vi "Meas_monitordata_struct_Add.vi"(1 "Active Sensors":bool[](array[boolean]), 2 "chk2scan":bool, 5 "Controls[]":refnum<vi>[](array[refnum]), 7 "Meas_monitordata_struct输入":refnum<k24>[](array[refnum]), 11 "错误输入（无错误）":errorcluster, 12 "sweep_count":i32, 13 "Meas_rang":i32[](array[numeric])) -> (6 "Meas_monitordata_struct输出":refnum<k24>[](array[refnum]), 15 "错误输出":errorcluster)   [LabVIEW 2017]
doc: "for measurement monitor data"
uses:
  D:/test/PDLSTS/LV_PDL_Sample/DLL/STSProcess.dll
  DLL/STSProcess.dll
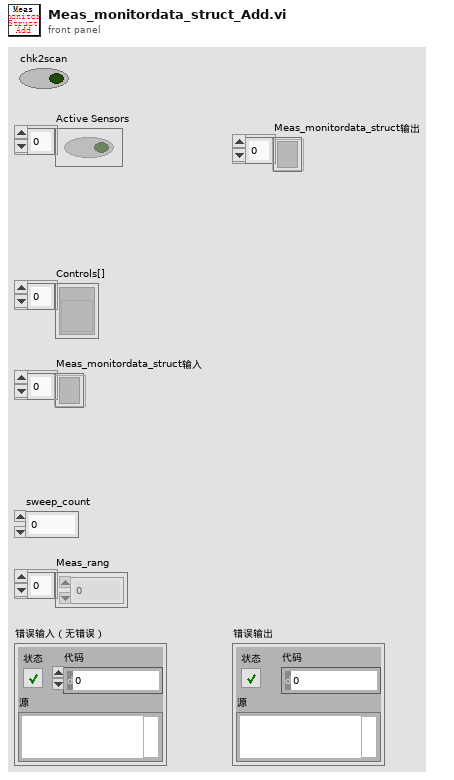
[diagram p1: front panel]
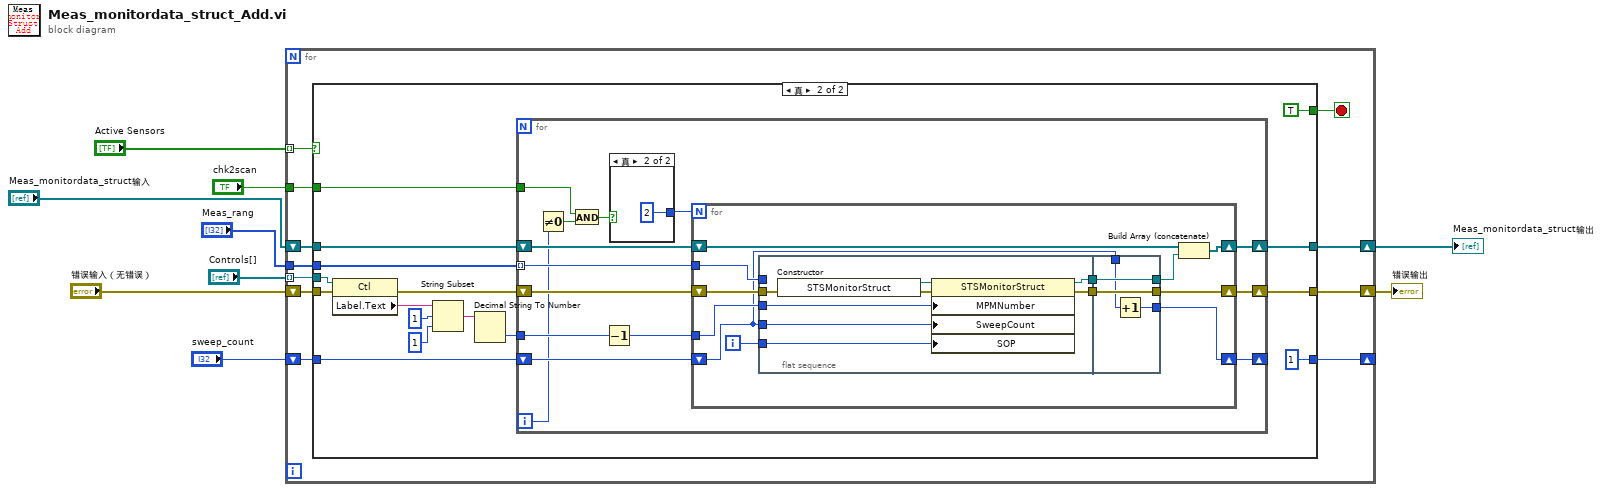
[diagram p0: block diagram]
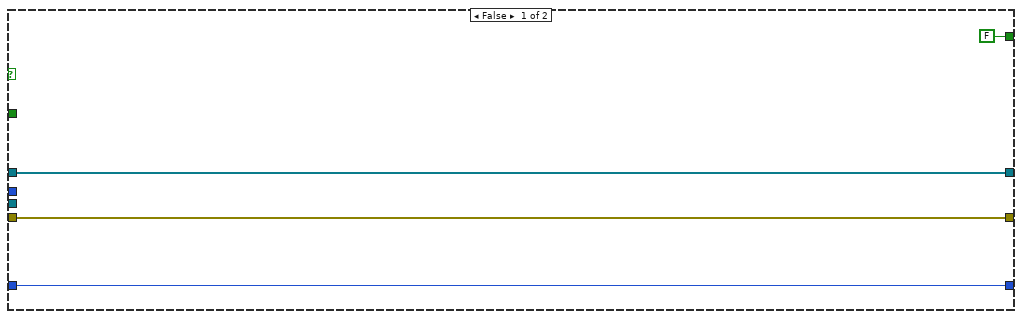
[diagram p2: hidden frame]
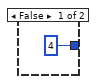
[diagram p3: hidden frame]
diagram:
  n1 = for {
    tunnel: "Active Sensors" -> [w20] mode=indexing
    tunnel: "Controls[]" -> [w19] mode=indexing
    tunnel: "Meas_rang" -> [w18]
    shift-right: [w16] -> w4
    shift-left: "Meas_monitordata_struct输入" -> [w17]
    shift-right: [w15] -> w6
    shift-left: "错误输入（无错误）" -> [w14]
    tunnel: "chk2scan" -> [w12]
    shift-right: [w10] -> _
    shift-left: "sweep_count" -> [w13]
    stop <- w11 stop-if-true
    n2 = case shown="真" w20 {
      tunnel: w19 -> [_ w40]
      tunnel: w17 -> [w24 w30]
      tunnel: [w24 w34] -> w16
      tunnel: [w23 w33] -> w15
      tunnel: w14 -> [w23 w32]
      tunnel: w18 -> [_ w31]
      tunnel: w13 -> [w21 w28]
      tunnel: w12 -> [_ w27]
      tunnel: [FALSE TRUE] -> w11
      tunnel: [w21 1] -> w10
      frame False {
      }
      frame True {
        n3 = property class="Ctl"(reference=w40, error in=w32) -> (error out=w29:errorcluster, "Label.Text"=w37:string)  [unwired: 1 out]
        n4 = String Subset(string=w37, offset (0)=1 ("偏移量(0)"), length (rest)=1 ("长度（剩余）")) -> (substring=w36:string)
        n5 = Decimal String To Number(string=w36) -> (number=w35:i32)  [unwired: 2 in, 1 out]
        n6 = for {
          tunnel: w35 -> [w54]
          tunnel: w31 -> [w50] mode=indexing
          shift-right: [w51] -> w33
          shift-left: w29 -> [w45]
          shift-right: [w53] -> w34
          shift-left: w30 -> [w46]
          tunnel: w27 -> [w43]
          shift-right: [w42] -> _
          shift-left: w28 -> [w44]
          i -> [w41]
          n7 = Not Equal To 0?(x=w41) -> (x != 0?=w49:bool)
          n8 = And(x=w43, y=w49) -> (x .and. y?=w48:bool)
          n9 = Decrement(x=w54) -> (x-1=w52:i32)
          n10 = case shown="真" w48 {
            tunnel: [4 2] -> w47
            frame False {
            }
            frame True {
            }
          }
          n11 = for {
            N: w47 -> [_]
            tunnel: w52 -> [w63]
            tunnel: w50 -> [w61]
            shift-right: [w62] -> w51
            shift-left: w45 -> [w57]
            shift-right: [w64] -> w53
            shift-left: w46 -> [w66]
            shift-right: [w55] -> w42
            shift-left: w44 -> [w56]
            i -> [w60]
            n12 = flat-sequence {
              tunnel: w63 -> [w69]
              tunnel: w61 -> [_]
              tunnel: w60 -> [w68]
              tunnel: [w72] -> w59
              tunnel: [w71] -> w58
              tunnel: w57 -> [w70]
              tunnel: w56 -> [w67]
              tunnel: [w77] -> w62
              tunnel: [w78] -> w65
              tunnel: w59 -> [w78]
              tunnel: w58 -> [w77]
              tunnel: [w76] -> w55
              tunnel: w56 -> [w75]
              frame #0 {
                n13 = constructor class="STSMonitorStruct"(error in=w70) -> (reference out=w74:refnum<k24>, error out=w73:errorcluster)  [unwired: 2 in, 1 out]
                n14 = property on="属性节点" class="STSMonitorStruct"(reference=w74, error in=w73, "MPMNumber"=w69, "SweepCount"=w67, "SOP"=w68) -> (reference out=w72:refnum<k24>, error out=w71:errorcluster)
              }
              frame #1 {
                n15 = Increment(x=w75) -> (x+1=w76:i32)
              }
            }
            n16 = Build Array (concatenate)(w66, w65) -> (w64:refnum<k24>[])
          }
        }
      }
    }
  }
  "错误输出" <- w6
  "Meas_monitordata_struct输出" <- w4
